vi "Drive 6.vi"(6 "Rotation":dbl, 7 "Gyro Angle":dbl, 8 "error in (no error)":errorcluster, 9 "Y":dbl, 10 "X":dbl, 11 "RobotDriveDevRef 2":T1={"DevStatus"={"status"=FALSE, "code"=0, "source"=""}, "Motors[]"=[], "Square Inputs"=FALSE, "Max Output"=1.0, "Isochronous"=FALSE}) -> (0 "error out":errorcluster, 1 "Current":dbl[](array[numeric]), 2 "Motor Values":dbl[](array[numeric]), 3 "RobotDriveDevRef":T1={"DevStatus"={"status"=FALSE, "code"=0, "source"=""}, "Motors[]"=[], "Square Inputs"=FALSE, "Max Output"=1.0, "Isochronous"=FALSE})   [LabVIEW 2013]
uses:
  <vilib>/Rock Robotics/SystemInterfaces/NetworkCommunication/NetComm_UsageReport_ResourceType.ctl
  <vilib>/Rock Robotics/WPI/CAN/Jaguar/SubVIs/WPI_CANJaguar_StatusSelect.ctl
  <vilib>/Rock Robotics/WPI/PWM/WPI_PWMTransform_ConPane.ctl
  <vilib>/Rock Robotics/SystemInterfaces/Typedef/FPGA_TypedefDigitalModule.ctl
  <vilib>/Rock Robotics/SystemInterfaces/DIO/FPGA_DIOPWMChannel.ctl
  <vilib>/Rock Robotics/WPI/PWM/WPI_PWMDeadband.ctl
  <vilib>/Rock Robotics/WPI/CAN/Jaguar/SubVIs/WPI_CANJaguar_ControlMode.ctl
  <vilib>/Rock Robotics/WPI/MotorControl/WPI_MotorControlDeviceRef.ctl
  <vilib>/Rock Robotics/WPI/RobotDrive/WPI_RobotDriveDevRef.ctl
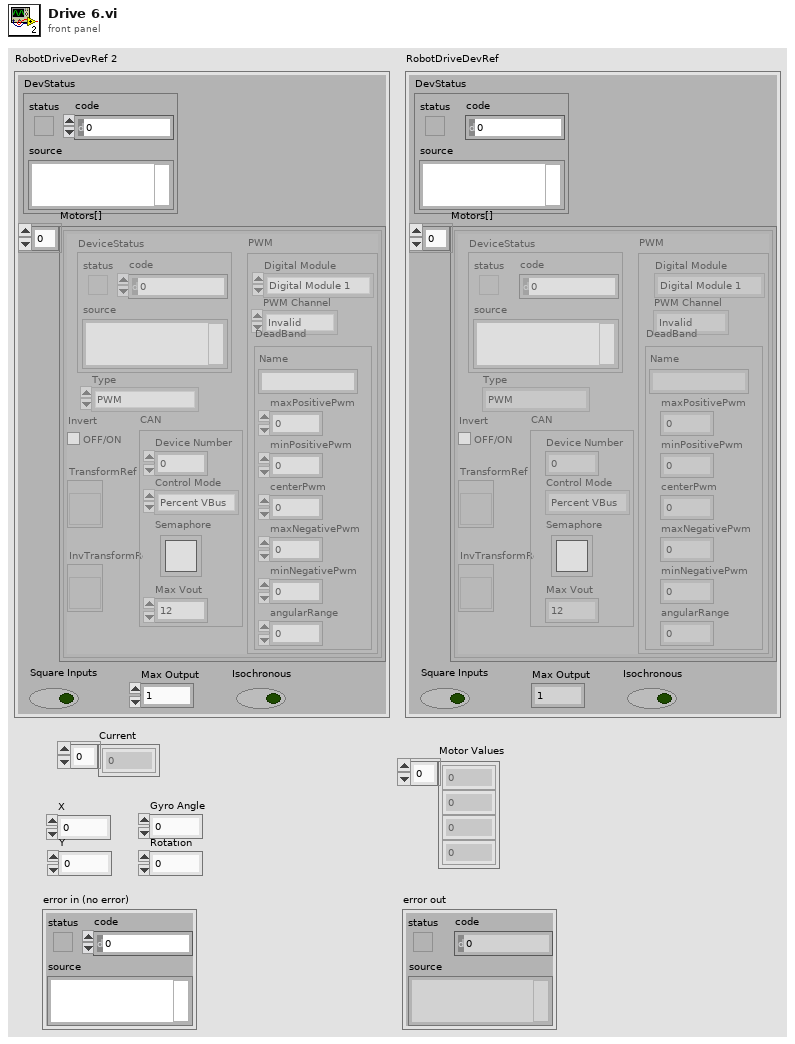
[diagram p1: front panel]
types:
  T1 = typedef "WPI_RobotDriveDevRef.ctl" = cluster{"DevStatus":errorcluster, "Motors[]":T2[], "Square Inputs":bool, "Max Output":dbl, "Isochronous":bool}
  T2 = typedef "WPI_MotorControlDeviceRef.ctl" = cluster{"DeviceStatus":errorcluster, "Type":enum16{"PWM", "CAN"}, "PWM":cluster{"Digital Module":T3, "PWM Channel":T4, "DeadBand":T5}, "CAN":cluster{"Device Number":u8, "Control Mode":T6, "Semaphore":T7, "Max Vout":dbl}, "Invert":bool, "TransformRef":T8, "InvTransformRef":T8}
  T3 = typedef "FPGA_TypedefDigitalModule.ctl" = enum16{"Digital Module 1", "Digital Module 2"}
  T4 = typedef "FPGA_DIOPWMChannel.ctl" = enum8{"PWM 1", "PWM 2", "PWM 3", "PWM 4", "PWM 5", "PWM 6", "PWM 7", "PWM 8", "PWM 9", "PWM 10", "Invalid"}
  T5 = typedef "WPI_PWMDeadband.ctl" = cluster{"Name":string, "maxPositivePwm":i32, "minPositivePwm":i32, "centerPwm":i32, "maxNegativePwm":i32, "minNegativePwm":i32, "angularRange":u16}
  T6 = typedef "WPI_CANJaguar_ControlMode.ctl" = enum8{"Percent VBus", "Current", "Speed", "Position", "Voltage"}
  T7 = typedef "Semaphore RefNum" = refnum<k1>
  T8 = typedef "WPI_PWMTransform_ConPane.ctl" = refnum<vi>
  T9 = typedef "NetComm_UsageReport_ResourceType.ctl" = enum8{"Controller", "Module", "Language", "CANPlugin", "Accelerometer", "ADXL345", "AnalogChannel", "AnalogTrigger", "AnalogTriggerOutput", "CANJaguar", "Compressor", "Counter", "Dashboard", "DigitalInput", "DigitalOutput", "DriverStationCIO", "DriverStationEIO", "DriverStationLCD", "Encoder", "GearTooth", "Gyro", "I2C", "Framework", "Jaguar", "Joystick", "Kinect", "KinectStick", "PIDController", "Preferences", "PWM", "Relay", "RobotDrive", "SerialPort", "Servo", "Solenoid", "SPI", "Task", "Ultrasonic", "Victor", "Button", "Command", "AxisCamera", "PCVideoServer", "SmartDashboard", "Talon", "HiTechnicColorSensor", "HiTechnicAccel", "HiTechnicCompass", "SRF08"}
  T10 = typedef "WPI_CANJaguar_StatusSelect.ctl" = enum16{"Output Percent VBus", "Output Voltage", "Bus Voltage", "Current", "Temperature", "Position", "Speed", "Limit Switches", "Faults", "Fault Counters", "Power Cycle"}
  T11 = typedef "WPI_CANJaguar_Status.ctl" = cluster{"Output Percent VBus":dbl, "Output Voltage":dbl, "Bus Voltage":dbl, "Current":dbl, "Temperature":dbl, "Position":dbl, "Speed":dbl, "Limits":cluster{"Forward Limit":bool, "Reverse Limit":bool, "Forward Soft Limit":bool, "Reverse Soft Limit":bool, "Sticky Forward Limit":bool, "Sticky Reverse Limit":bool, "Sticky Forward Soft Limit":bool, "Sticky Reverse Soft Limit":bool}, "Faults":cluster{"Current Fault":bool, "Temperature Fault":bool, "Bus Voltage Fault":bool, "Gate Driver Fault":bool, "Comm Fault":bool}, "Fault Counters":cluster{"Current Faults":u8, "Temperature Faults":u8, "Bus Voltage Faults":u8, "Gate Driver Faults":u8, "Comm Faults":u8, "CAN Status":u8, "CAN RX Errors":u8, "CAN TX Errors":u8}, "Power Cycle":bool}
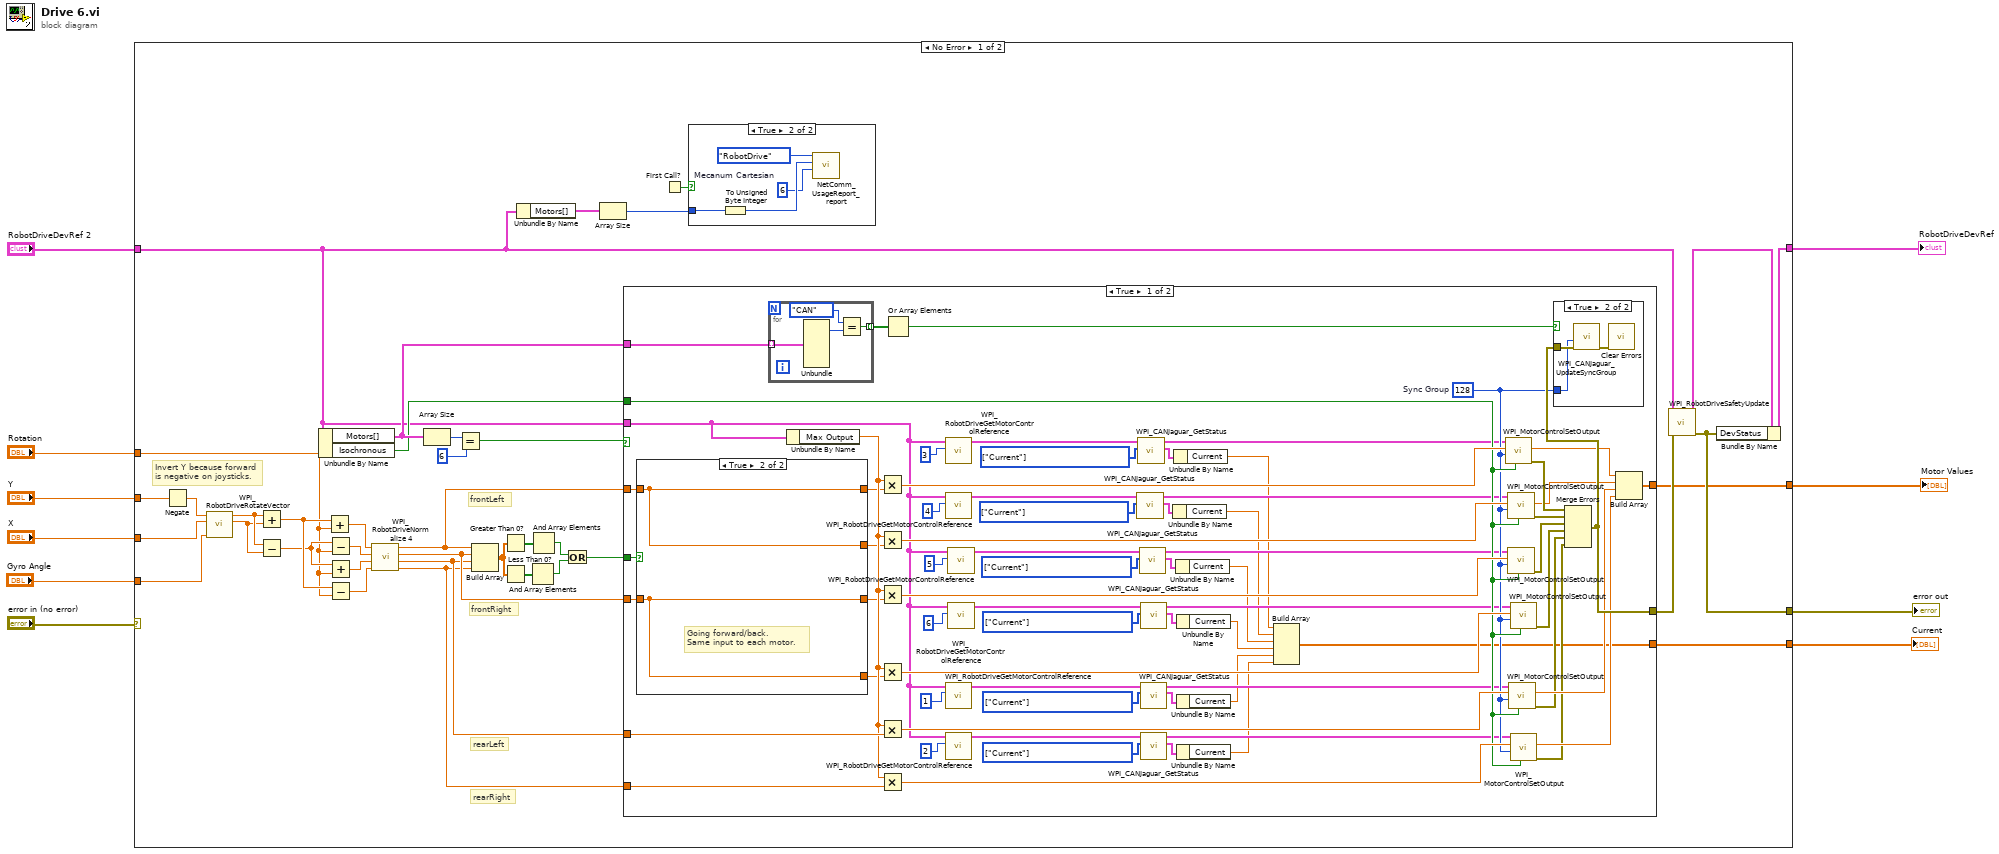
[diagram p0: block diagram]
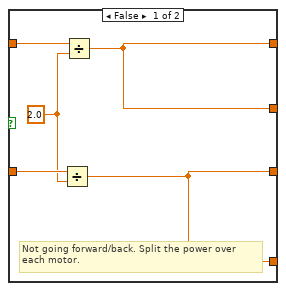
[diagram p3: hidden frame]
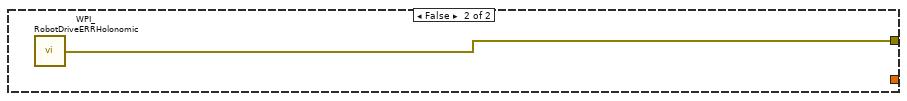
[diagram p5: hidden frame]
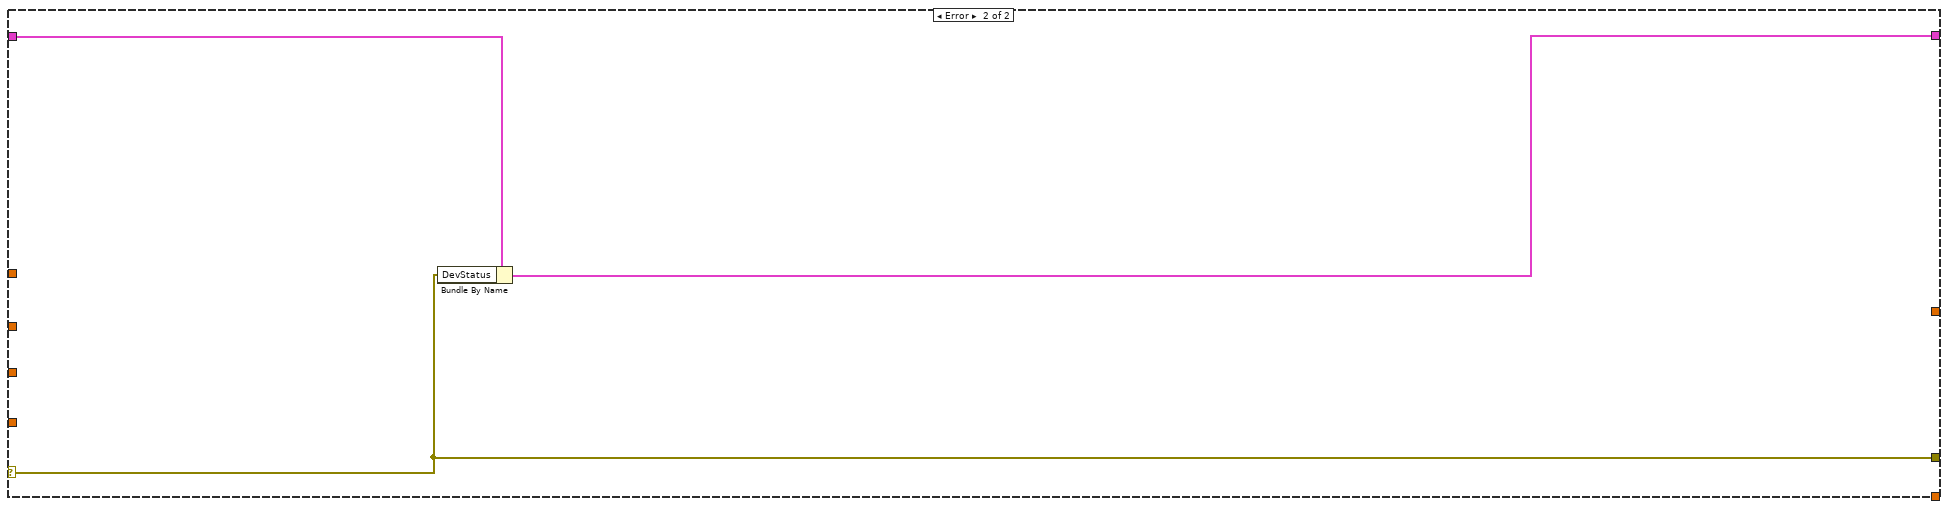
[diagram p6: hidden frame]
diagram:
  n1 = case shown="No Error" "error in (no error)" {
    selector: "error in (no error)" -> [_ w139]
    tunnel: "Y" -> [w34 _]
    tunnel: "X" -> [w35 _]
    tunnel: "RobotDriveDevRef 2" -> [w23 w141]
    tunnel: [w45 w140] -> w6
    tunnel: [w29 w139] -> w5
    tunnel: "Rotation" -> [w36 _]
    tunnel: "Gyro Angle" -> [w33 _]
    tunnel: [w22 _] -> w2
    tunnel: [w11 _] -> w1
    frame No Error {
      # "Invert Y because forward is negative on joysticks."
      # "rearLeft"
      # "frontRight"
      # "rearRight"
      # "frontLeft"
      n2 = Negate(x=w34) -> (-x=w32:dbl)
      n3 = call <vilib>:"WPI_RobotDriveRotateVector.vi"("Angle"=w33, "X"=w35, "Y"=w32) -> ("X'"=w43:dbl, "Y'"=w44:dbl)  [unwired: 7 out]
      n4 = Add(x=w44, y=w43) -> (x+y=w41:dbl)
      n5 = Subtract(x=w44, y=w43) -> (x-y=w39:dbl)
      n6 = Unbundle By Name(w23) -> ("Motors[]"=w28:T2[], "Isochronous"=w27:bool)
      n7 = Add(x=w41, y=w36) -> (x+y=w37:dbl)
      n8 = Subtract(x=w39, y=w36) -> (x-y=w38:dbl)
      n9 = Add(x=w39, y=w36) -> (x+y=w40:dbl)
      n10 = Subtract(x=w41, y=w36) -> (x-y=w42:dbl)
      n11 = call <vilib>:"WPI_RobotDriveNormalize 4.vi"("D"=w42, "C"=w40, "B"=w38, "A"=w37) -> ("D'"=w18:dbl, "C'"=w19:dbl, "B'"=w20:dbl, "A'"=w21:dbl)
      n12 = Array Size(array=w28) -> (size(s)=w48:i32)
      n13 = Equal?(x=w48, y=6) -> (x = y?=w46:bool)
      n14 = Build Array(w21, w20, w19, w18) -> (w17:dbl[])
      n15 = Greater Than 0?(x=w17) -> (x > 0?=w16:bool[])
      n16 = Less Than 0?(x=w17) -> (x < 0?=w15:bool[])
      n17 = Unbundle By Name(w23) -> ("Motors[]"=w25:T2[])
      n18 = And Array Elements(Boolean array=w15) -> (logical AND=w13:bool)
      n19 = And Array Elements(Boolean array=w16) -> (logical AND=w14:bool)
      n20 = Or(x=w14, y=w13) -> (x .or. y?=w12:bool)
      n21 = Array Size(array=w25) -> (size(s)=w24:i32)
      n22 = case shown="True" w46 {
        tunnel: w21 -> [w90 _]
        tunnel: w20 -> [w89 _]
        tunnel: w23 -> [w104 _]
        tunnel: [w112 w138] -> w31
        tunnel: w19 -> [w123 _]
        tunnel: w18 -> [w122 _]
        tunnel: w28 -> [w113 _]
        tunnel: w27 -> [w103 _]
        tunnel: [w110 _] -> w22
        tunnel: w12 -> [w84 _]
        tunnel: [w53 _] -> w11
        frame True {
          w71 = T10[] [enum."Current"] items=["Output Percent VBus", "Output Voltage", "Bus Voltage", "Current", "Temperature", "Position", "Speed", "Limit Switches", "Faults", "Fault Counters", "Power Cycle"] ("Status Select")
          w73 = T10[] [enum."Current"] items=["Output Percent VBus", "Output Voltage", "Bus Voltage", "Current", "Temperature", "Position", "Speed", "Limit Switches", "Faults", "Fault Counters", "Power Cycle"] ("Status Select")
          w75 = T10[] [enum."Current"] items=["Output Percent VBus", "Output Voltage", "Bus Voltage", "Current", "Temperature", "Position", "Speed", "Limit Switches", "Faults", "Fault Counters", "Power Cycle"] ("Status Select")
          w77 = T10[] [enum."Current"] items=["Output Percent VBus", "Output Voltage", "Bus Voltage", "Current", "Temperature", "Position", "Speed", "Limit Switches", "Faults", "Fault Counters", "Power Cycle"] ("Status Select")
          w79 = T10[] [enum."Current"] items=["Output Percent VBus", "Output Voltage", "Bus Voltage", "Current", "Temperature", "Position", "Speed", "Limit Switches", "Faults", "Fault Counters", "Power Cycle"] ("Status Select")
          w83 = T10[] [enum."Current"] items=["Output Percent VBus", "Output Voltage", "Bus Voltage", "Current", "Temperature", "Position", "Speed", "Limit Switches", "Faults", "Fault Counters", "Power Cycle"] ("Status Select")
          w102 = u8 128  # Sync Group
          n23 = case shown="True" w84 {
            tunnel: w90 -> [w128 w129]
            tunnel: w89 -> [w127 w130]
            tunnel: [w125 w130] -> w88
            tunnel: [w125 w130] -> w87
            tunnel: [w124 w129] -> w86
            tunnel: [w124 w129] -> w85
            frame False {
              w126 = 2.0 ("y")
              # "Not going forward/back. Split the power over\neach motor."
              n24 = Divide(x=w127, y=w126) -> (x/y=w125:dbl)
              n25 = Divide(x=w128, y=w126) -> (x/y=w124:dbl)
            }
            frame True {
              # "Going forward/back.\nSame input to each motor."
            }
          }
          n26 = for {
            tunnel: w113 -> [w134] mode=indexing
            tunnel: [w131] -> w114 mode=indexing
            n27 = Unbundle(w134) -> ("Type"=w133:enum16{"PWM", "CAN"})  [unwired: 6 out]
            n28 = Equal?(x=enum16{"PWM", "CAN"}."CAN" ("Type"), y=w133) -> (x = y?=w131:bool)
          }
          n29 = Unbundle By Name(w104) -> ("Max Output"=w95:dbl)
          n30 = Multiply(x=w95, y=w86) -> (x*y=w121:dbl)
          n31 = Multiply(x=w95, y=w85) -> (x*y=w120:dbl)
          n32 = Multiply(x=w95, y=w87) -> (x*y=w106:dbl)
          n33 = Multiply(x=w95, y=w88) -> (x*y=w105:dbl)
          n34 = Multiply(x=w95, y=w123) -> (x*y=w119:dbl)
          n35 = Multiply(x=w95, y=w122) -> (x*y=w118:dbl)
          n36 = Or Array Elements(Boolean array=w114) -> (logical OR=w115:bool)
          n37 = call <vilib>:"WPI_RobotDriveGetMotorControlReference.vi"("MotorIndex"=3, "RobotDriveDevRef"=w104) -> ("MotorControlDeviceRef"=w82:T2)  [unwired: 9 out]
          n38 = call <vilib>:"WPI_RobotDriveGetMotorControlReference.vi"("MotorIndex"=4, "RobotDriveDevRef"=w104) -> ("MotorControlDeviceRef"=w69:T2)  [unwired: 9 out]
          n39 = call <vilib>:"WPI_RobotDriveGetMotorControlReference.vi"("MotorIndex"=1, "RobotDriveDevRef"=w104) -> ("MotorControlDeviceRef"=w63:T2)  [unwired: 9 out]
          n40 = call <vilib>:"WPI_RobotDriveGetMotorControlReference.vi"("MotorIndex"=2, "RobotDriveDevRef"=w104) -> ("MotorControlDeviceRef"=w61:T2)  [unwired: 9 out]
          n41 = call <vilib>:"WPI_RobotDriveGetMotorControlReference.vi"("MotorIndex"=5, "RobotDriveDevRef"=w104) -> ("MotorControlDeviceRef"=w67:T2)  [unwired: 9 out]
          n42 = call <vilib>:"WPI_RobotDriveGetMotorControlReference.vi"("MotorIndex"=6, "RobotDriveDevRef"=w104) -> ("MotorControlDeviceRef"=w65:T2)  [unwired: 9 out]
          n43 = call <vilib>:"WPI_CANJaguar_GetStatus.vi"("Status Select"=w79, "CAN Jaguar Ref"=w69) -> ("Status"=w78:T11, "CAN Jaguar Ref Out"=w68:T2)  [unwired: 7 in, 1 out]
          n44 = call <vilib>:"WPI_CANJaguar_GetStatus.vi"("Status Select"=w83, "CAN Jaguar Ref"=w82) -> ("Status"=w80:T11, "CAN Jaguar Ref Out"=w81:T2)  [unwired: 7 in, 1 out]
          n45 = call <vilib>:"WPI_CANJaguar_GetStatus.vi"("Status Select"=w77, "CAN Jaguar Ref"=w67) -> ("Status"=w76:T11, "CAN Jaguar Ref Out"=w66:T2)  [unwired: 7 in, 1 out]
          n46 = call <vilib>:"WPI_CANJaguar_GetStatus.vi"("Status Select"=w75, "CAN Jaguar Ref"=w65) -> ("Status"=w74:T11, "CAN Jaguar Ref Out"=w64:T2)  [unwired: 7 in, 1 out]
          n47 = call <vilib>:"WPI_CANJaguar_GetStatus.vi"("Status Select"=w73, "CAN Jaguar Ref"=w63) -> ("Status"=w72:T11, "CAN Jaguar Ref Out"=w62:T2)  [unwired: 7 in, 1 out]
          n48 = call <vilib>:"WPI_CANJaguar_GetStatus.vi"("Status Select"=w71, "CAN Jaguar Ref"=w61) -> ("Status"=w70:T11, "CAN Jaguar Ref Out"=w60:T2)  [unwired: 7 in, 1 out]
          n49 = Unbundle By Name(w78) -> ("Current"=w58:dbl)
          n50 = Unbundle By Name(w80) -> ("Current"=w59:dbl)
          n51 = Unbundle By Name(w76) -> ("Current"=w57:dbl)
          n52 = Unbundle By Name(w74) -> ("Current"=w56:dbl)
          n53 = Unbundle By Name(w72) -> ("Current"=w55:dbl)
          n54 = Unbundle By Name(w70) -> ("Current"=w54:dbl)
          n55 = Build Array(w59, w58, w57, w56, w55, w54) -> (w53:dbl[])
          n56 = call <vilib>:"WPI_MotorControlSetOutput.vi"("Isochronous"=w103, "Sync Group"=w102, "Output"=w121, "MotorControlDevRef"=w81) -> ("error out"=w116:errorcluster, "Motor Output"=w111:dbl)  [unwired: 1 in, 5 out]
          n57 = call <vilib>:"WPI_MotorControlSetOutput.vi"("Isochronous"=w103, "Sync Group"=w102, "Output"=w120, "MotorControlDevRef"=w68) -> ("error out"=w117:errorcluster, "Motor Output"=w109:dbl)  [unwired: 1 in, 5 out]
          n58 = call <vilib>:"WPI_MotorControlSetOutput.vi"("Isochronous"=w103, "Sync Group"=w102, "Output"=w106, "MotorControlDevRef"=w66) -> ("error out"=w94:errorcluster)  [unwired: 1 in, 6 out]
          n59 = call <vilib>:"WPI_MotorControlSetOutput.vi"("Isochronous"=w103, "Sync Group"=w102, "Output"=w119, "MotorControlDevRef"=w62) -> ("error out"=w92:errorcluster, "Motor Output"=w108:dbl)  [unwired: 1 in, 5 out]
          n60 = call <vilib>:"WPI_MotorControlSetOutput.vi"("Isochronous"=w103, "Sync Group"=w102, "Output"=w105, "MotorControlDevRef"=w64) -> ("error out"=w93:errorcluster)  [unwired: 1 in, 6 out]
          n61 = call <vilib>:"WPI_MotorControlSetOutput.vi"("Isochronous"=w103, "Sync Group"=w102, "Output"=w118, "MotorControlDevRef"=w60) -> ("error out"=w91:errorcluster, "Motor Output"=w107:dbl)  [unwired: 1 in, 5 out]
          n62 = Merge Errors(w116, w117, w94, w93, w92, w91) -> (w112:errorcluster)
          n63 = case shown="True" w115 {
            tunnel: w112 -> [_ w136]
            tunnel: w102 -> [_ w135]
            frame False {
            }
            frame True {
              n64 = call <vilib>:"WPI_CANJaguar_UpdateSyncGroup.vi"("error in (no error)"=w136, "Sync Group"=w135) -> ("error out"=w137:errorcluster)  [unwired: 9 out]
              n65 = call <vilib>:"Clear Errors.vi"("error in (no error)"=w137) -> ()  [unwired: 7 out]
            }
          }
          n66 = Build Array(w111, w109, w108, w107) -> (w110:dbl[])
        }
        frame False {
          n67 = call <vilib>:"WPI_RobotDriveERRHolonomic.vi"() -> ("error out"=w138:errorcluster)
        }
      }
      n68 = First Call?() -> (First Call?: T/F=w26:bool)
      n69 = case shown="True" w26 {
        tunnel: w24 -> [_ w51]
        frame False {
        }
        frame True {
          w49 = u8 6  # Mecanum Cartesian
          n70 = To Unsigned Byte Integer(number=w51) -> (unsigned 8bit integer=w50:u8)
          n71 = call <vilib>:"NetComm_UsageReport_report.vi"("Context"=w49, "Instance Number"=w50, "Resource Type"=NetComm_UsageReport_ResourceType."RobotDrive") -> ()  [unwired: 9 in]
        }
      }
      n72 = call <vilib>:"WPI_RobotDriveSafetyUpdate.vi"("error in (no error)"=w31, "RobotDriveDevRef"=w23) -> ("error out"=w29:errorcluster, "RobotDriveDevRef"=w30:T1)  [unwired: 8 out]
      n73 = Bundle By Name(cluster=w30, "DevStatus"=w29) -> (w45:T1)
    }
    frame Error {
      n74 = Bundle By Name(cluster=w141, "DevStatus"=w139) -> (w140:T1)
    }
  }
  "error out" <- w5
  "RobotDriveDevRef" <- w6
  "Motor Values" <- w2
  "Current" <- w1
